vi "reset.vi"(8 "error in (no error)":errorcluster, 11 "Status Actor in":refnum<class "Status Actor.lvclass">) -> (0 "error out":errorcluster, 3 "Status Actor out":refnum<class "Status Actor.lvclass">)   [LabVIEW 2019, in "Status Actor.lvlib" / "Status Actor.lvclass"]
uses:
  Status Actor.lvclass
  <vilib>/event_ctls.llb/usereventprio.ctl
  Status Actor.lvclass/Status Actor.ctl
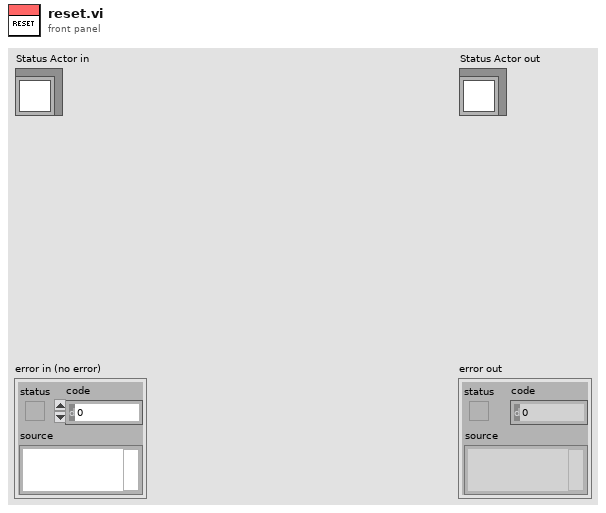
[diagram p1: front panel]
types:
  T1 = typedef "usereventprio.ctl" = enum32{"high priority", "normal priority"}
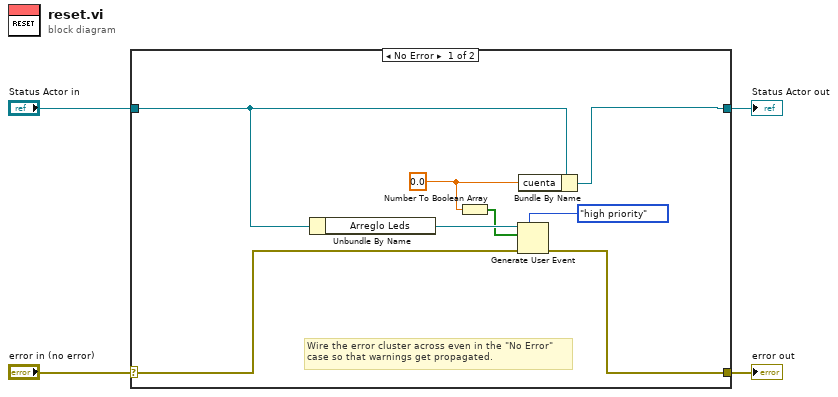
[diagram p0: block diagram]
diagram:
  n1 = case shown="No Error" "error in (no error)" {
    selector: "error in (no error)" -> [w7 w14]
    tunnel: [w6 w14] -> w3
    tunnel: [w11 w13] -> w1
    tunnel: "Status Actor in" -> [w10 w13]
    frame No Error {
      w9 = 0.0 ("Cuenta")
      # "Wire the error cluster across even in the \"No Error\"\ncase so that warnings get propagated."
      n2 = Unbundle By Name(w10) -> ("Arreglo Leds"=w12:refnum<user-event>)
      n3 = Number To Boolean Array(number=w9) -> (Boolean array=w8:bool[])
      n4 = Generate User Event(priority (normal)=usereventprio."high priority", user event=w12, event data cluster=w8, error in=w7) -> (error out=w6:errorcluster)  [unwired: 1 out]
      n5 = Bundle By Name(cluster=w10, "cuenta"=w9) -> (w11:refnum<class "Status Actor.lvclass">)
    }
    frame Error {
    }
  }
  "error out" <- w3
  "Status Actor out" <- w1
